vi "CRYCalc worst fit of average.vi"(7 "Step Setup VI No":i32, 9 "rank number(worst curve)":i32, 11 "Data in":T1 {"Z data" items=["dB", "Lin"]; "X data" items=["dB", "Lin"]; "Y data" items=["dB", "Lin"]; "Z dB ref" format="%.1f"; "Z axis" items=["Log", "Lin"]; "X dB ref" format="%.1f"; "X axis" items=["Log", "Lin"]; "Y axis" items=["Log", "Lin"]; "Y dB ref" format="%.1f"; "Curve"."z" format="%.2f"; "Curve"."y" format="%.2f"; "Curve"."x" format="%.2f"}) -> (3 "Worst Fit Out":T1 {"Z data" items=["dB", "Lin"]; "X data" items=["dB", "Lin"]; "Y data" items=["dB", "Lin"]; "Z dB ref" format="%.1f"; "Z axis" items=["Log", "Lin"]; "X dB ref" format="%.1f"; "X axis" items=["Log", "Lin"]; "Y axis" items=["Log", "Lin"]; "Y dB ref" format="%.1f"; "Curve"."z" format="%.2f"; "Curve"."y" format="%.2f"; "Curve"."x" format="%.2f"})   [LabVIEW 2013]
uses:
  Typedef Control/CRYData Cluster Array.ctl
  Typedef Control/CRYData Cluster.ctl
  <vilib>/Analysis/NI_AALBase.lvlib
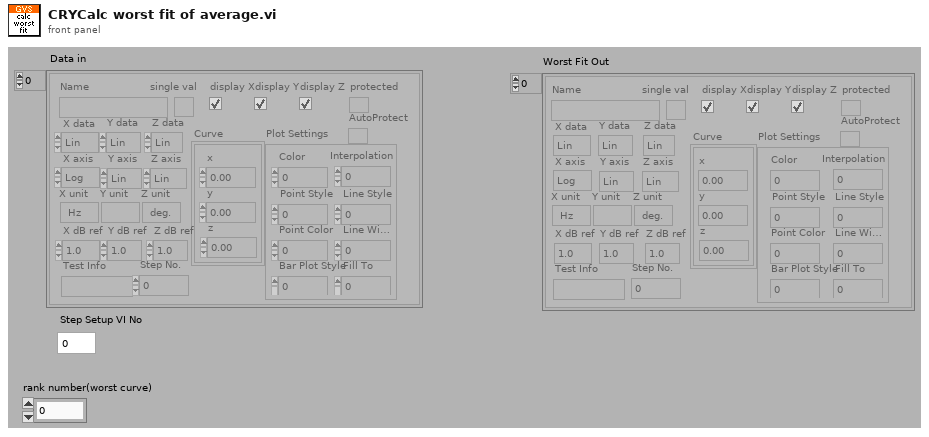
[diagram p1: front panel]
types:
  T1 = typedef "CRYData Cluster Array.ctl" = T2[]
  T2 = typedef "CRYData Cluster.ctl" = cluster{"Name":string, "Curve":cluster{"x":dbl, "y":dbl, "z":dbl}[], "X data":u16, "Y data":u16, "Z data":u16, "X axis":u16, "Y axis":u16, "Z axis":u16, "X unit":string, "Y unit":string, "Z unit":string, "X dB ref":dbl, "Y dB ref":dbl, "Z dB ref":dbl, "single val":bool, "protected":bool, "display X":bool, "display Y":bool, "display Z":bool, "Test Info":string, "Step No.":i32, "Plot Settings":cluster{"Color":u32, "Interpolation":u8, "Point Style":u8, "Line Style":u8, "Point Color":u32, "Line Width":u8, "Bar Plot Style":u8, "Fill To":i16}, "AutoProtect":bool}
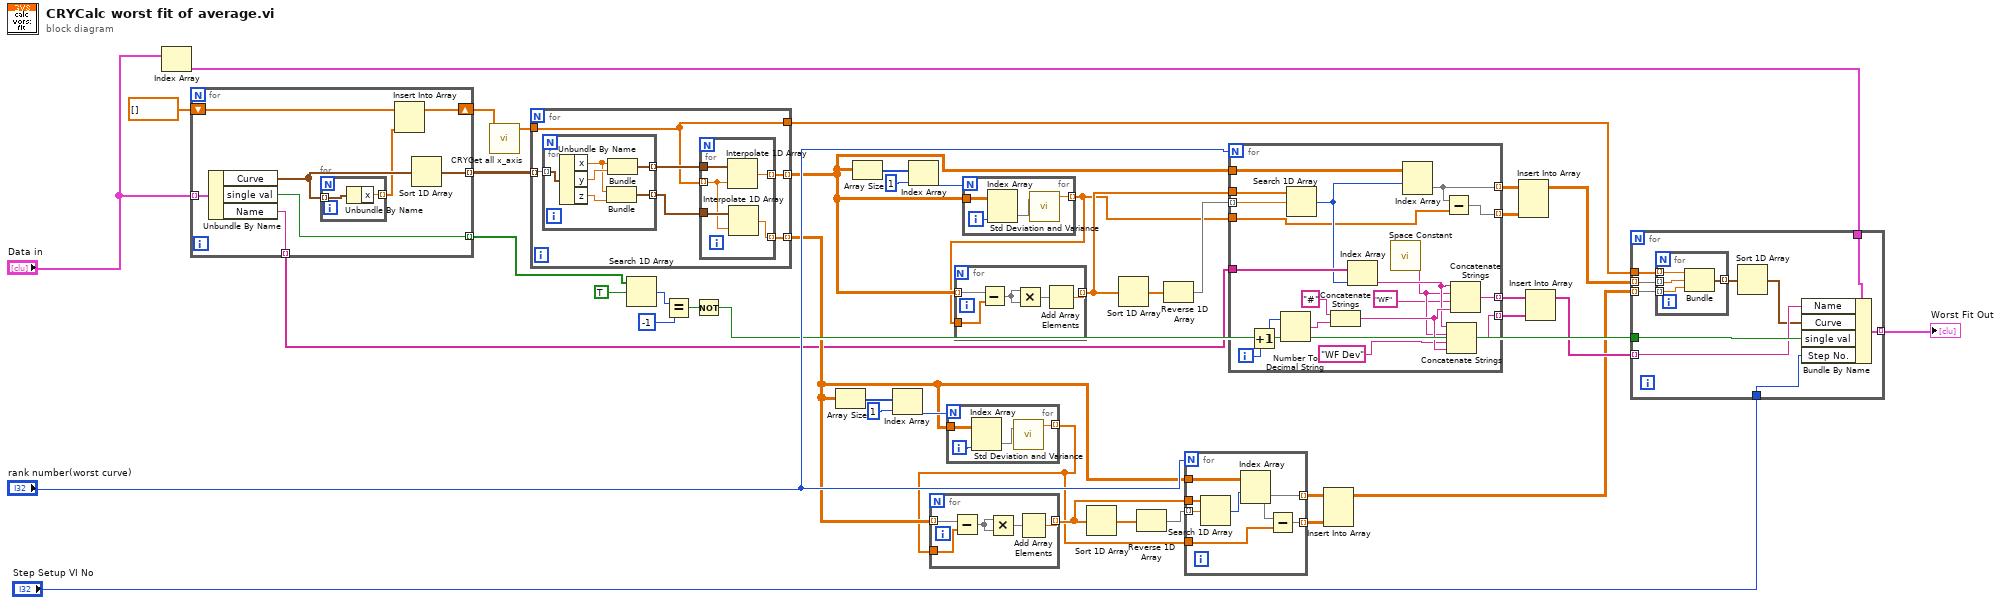
[diagram p0: block diagram]
diagram:
  n1 = Index Array(array="Data in") -> (element=w39:T2)  [unwired: 1 in]
  n2 = for {
    tunnel: [w43] -> w35 mode=indexing
    tunnel: "Data in" -> [w45] mode=indexing
    shift-right: [w48] -> w15
    shift-left: dbl[] [] ("x_Array") -> [w47]
    tunnel: [w46] -> w37 mode=indexing
    tunnel: [w44] -> w2 mode=indexing
    n3 = Unbundle By Name(w45) -> ("Curve"=w50:cluster{"x":dbl, "y":dbl, "z":dbl}[], "single val"=w46:bool, "Name"=w44:string)
    n4 = for {
      tunnel: w50 -> [w51] mode=indexing
      tunnel: [w52] -> w49 mode=indexing
      n5 = Unbundle By Name(w51) -> ("x"=w52:dbl)
    }
    n6 = Insert Into Array(array=w47, new element=w49) -> (w48:dbl[])  [unwired: 1 in]
    n7 = Sort 1D Array(array=w50) -> (sorted array=w43:cluster{"x":dbl, "y":dbl, "z":dbl}[])
  }
  n8 = call "CRYGet all x_axis.vi"("x_Array in"=w15) -> ("X_axis out"=w34:dbl[])  [unwired: 1 in, 9 out]
  n9 = for {
    tunnel: w35 -> [w54] mode=indexing
    tunnel: [w58] -> w19 mode=indexing
    tunnel: w34 -> [w53]
    tunnel: [w53] -> w38
    tunnel: [w55] -> w6 mode=indexing
    n10 = for {
      tunnel: [w63] -> w57 mode=indexing
      tunnel: w54 -> [w62] mode=indexing
      tunnel: [w59] -> w56 mode=indexing
      n11 = Unbundle By Name(w62) -> ("x"=w60:dbl, "y"=w64:dbl, "z"=w61:dbl)
      n12 = Bundle("x"=w60, "z"=w61) -> (w59:cluster{"x":dbl, "z":dbl})  [unwired: 1 out]
      n13 = Bundle("x"=w60, "y"=w64) -> (w63:cluster{"x":dbl, "y":dbl})  [unwired: 1 out]
    }
    n14 = for {
      tunnel: [w69] -> w58 mode=indexing
      tunnel: w57 -> [w68]
      tunnel: w53 -> [w66] mode=indexing
      tunnel: w56 -> [w67]
      tunnel: [w65] -> w55 mode=indexing
      n15 = Interpolate 1D Array(1:w66, 2:w68) -> (0:w69:dbl)
      n16 = Interpolate 1D Array(1:w66, 2:w67) -> (0:w65:dbl)
    }
  }
  n17 = Search 1D Array(1D array=w37, element=TRUE) -> (index of element=w32:i32)  [unwired: 1 out]
  n18 = Equal?(x=w32, y=-1) -> (x = y?=w30:bool)
  n19 = Not(x=w30) -> (.not. x?=w29:bool)
  n20 = Array Size(array=w6) -> (size(s)=w11:i32[])
  n21 = Array Size(array=w19) -> (size(s)=w24:i32[])
  n22 = Index Array(array=w11, index=1) -> (element=w10:i32)
  n23 = Index Array(array=w24, index=1) -> (element=w25:i32)
  n24 = for {
    N: w10 -> [_]
    tunnel: w6 -> [w73]
    tunnel: [w71] -> w3 mode=indexing
    i -> [w70]
    n25 = Index Array(array=w73, index (col)=w70) -> (element=w72:dbl[])  [unwired: 1 in]
    n26 = call <vilib>:"Std Deviation and Variance.vi"("X"=w72) -> ("mean"=w71:dbl)  [unwired: 1 in, 2 out]
  }
  n27 = for {
    tunnel: w6 -> [w74] mode=indexing
    tunnel: w3 -> [w77]
    tunnel: [w78] -> w8 mode=indexing
    n28 = Subtract(x=w74, y=w77) -> (x-y=w75:dbl[])
    n29 = Multiply(x=w75, y=w75) -> (x*y=w76:dbl[])
    n30 = Add Array Elements(numeric array=w76) -> (sum=w78:dbl)
  }
  n31 = for {
    N: w25 -> [_]
    tunnel: w19 -> [w82]
    tunnel: [w80] -> w4 mode=indexing
    i -> [w79]
    n32 = Index Array(array=w82, index (col)=w79) -> (element=w81:dbl[])  [unwired: 1 in]
    n33 = call <vilib>:"Std Deviation and Variance.vi"("X"=w81) -> ("mean"=w80:dbl)  [unwired: 1 in, 2 out]
  }
  n34 = for {
    tunnel: w19 -> [w83] mode=indexing
    tunnel: w4 -> [w86]
    tunnel: [w87] -> w27 mode=indexing
    n35 = Subtract(x=w83, y=w86) -> (x-y=w84:dbl[])
    n36 = Multiply(x=w84, y=w84) -> (x*y=w85:dbl[])
    n37 = Add Array Elements(numeric array=w85) -> (sum=w87:dbl)
  }
  n38 = Sort 1D Array(array=w8) -> (sorted array=w9:dbl[])
  n39 = Sort 1D Array(array=w27) -> (sorted array=w26:dbl[])
  n40 = Reverse 1D Array(array=w9) -> (reversed array=w14:dbl[])
  n41 = Reverse 1D Array(array=w26) -> (reversed array=w16:dbl[])
  n42 = for {
    N: "rank number(worst curve)" -> [_]
    tunnel: w14 -> [w93] mode=indexing
    tunnel: w6 -> [w92]
    tunnel: w8 -> [w94]
    tunnel: [w90] -> w12 mode=indexing
    tunnel: [w88] -> w13 mode=indexing
    tunnel: w3 -> [w89]
    n43 = Search 1D Array(1D array=w94, element=w93) -> (index of element=w91:i32)  [unwired: 1 out]
    n44 = Index Array(array=w92, index (row)=w91) -> (element=w90:dbl[])  [unwired: 1 in]
    n45 = Subtract(x=w90, y=w89) -> (x-y=w88:dbl[])
  }
  n46 = for {
    N: "rank number(worst curve)" -> [_]
    tunnel: w16 -> [w112] mode=indexing
    tunnel: w19 -> [w111]
    tunnel: w27 -> [w113]
    tunnel: [w105] -> w23 mode=indexing
    tunnel: [w106] -> w22 mode=indexing
    tunnel: w2 -> [w110]
    tunnel: [w108] -> w20 mode=indexing
    tunnel: [w107] -> w21 mode=indexing
    tunnel: w4 -> [w104]
    i -> [w100]
    n47 = Increment(x=w100) -> (x+1=w101:i32)
    n48 = Number To Decimal String(number=w101) -> (decimal integer string=w102:string)  [unwired: 1 out]
    n49 = Search 1D Array(1D array=w113, element=w112) -> (index of element=w109:i32)  [unwired: 1 out]
    n50 = Concatenate Strings("#" ("string"), w102) -> (w99:string)
    n51 = Index Array(array=w110, index=w109) -> (element=w98:string)
    n52 = call <vilib>:"Space Constant.vi"() -> ("String"=w97:string)
    n53 = Index Array(array=w111, index (row)=w109) -> (element=w105:dbl[])  [unwired: 1 in]
    n54 = Subtract(x=w105, y=w104) -> (x-y=w106:dbl[])
    n55 = Concatenate Strings(w98, w97, "WF Dev" ("string"), w99) -> (w108:string)
    n56 = Concatenate Strings(w98, w97, "WF" ("string"), w99) -> (w107:string)
  }
  n57 = Insert Into Array(array=w12, new element=w13) -> (w5:dbl[][])  [unwired: 2 in]
  n58 = Insert Into Array(array=w23, new element=w22) -> (w17:dbl[][])  [unwired: 2 in]
  n59 = Insert Into Array(array=w21, new element=w20) -> (w18:string[])  [unwired: 1 in]
  n60 = for {
    tunnel: w38 -> [w123]
    tunnel: w5 -> [w122] mode=indexing
    tunnel: w29 -> [w121]
    tunnel: [w119] -> w42 mode=indexing
    tunnel: w18 -> [w118] mode=indexing
    tunnel: w17 -> [w117] mode=indexing
    tunnel: w39 -> [w116]
    tunnel: "Step Setup VI No" -> [w114]
    n61 = for {
      tunnel: w117 -> [w126] mode=indexing
      tunnel: [w127] -> w120 mode=indexing
      tunnel: w123 -> [w125] mode=indexing
      tunnel: w122 -> [w124] mode=indexing
      n62 = Bundle("x"=w125, w126, w124) -> (w127:cluster{"x":dbl, dbl, dbl})  [unwired: 1 out]
    }
    n63 = Sort 1D Array(array=w120) -> (sorted array=w115:cluster{"x":dbl, dbl, dbl}[])
    n64 = Bundle By Name(cluster=w116, "Name"=w118, "Curve"=w115, "single val"=w121, "Step No."=w114) -> (w119:T2)
  }
  "Worst Fit Out" <- w42
